vi "_UpdateUIDisplay.vi"(7 "Refs":T2, 9 "Action in":T1 caption="Action", 10 "Display State In in":T3 caption="State", 11 "Data In in":T6) -> (1 "Action out":T1 caption="Action", 2 "Display State In out":T3 caption="State", 3 "Data In out":T6)   [LabVIEW 2017, in "UI_TimeSelector.xctl"]
uses:
  UI_TimeSelector.xctl
  Data.ctl
  State.ctl
  Typedefs/INTERNAL-DATA.ctl
  Interface/DEF-Mode.ctl
  Typedefs/INTERNAL-REFs.ctl
  <vilib>/_xctls/Action.ctl
  <vilib>/_xctls/XControlSupport.lvlib
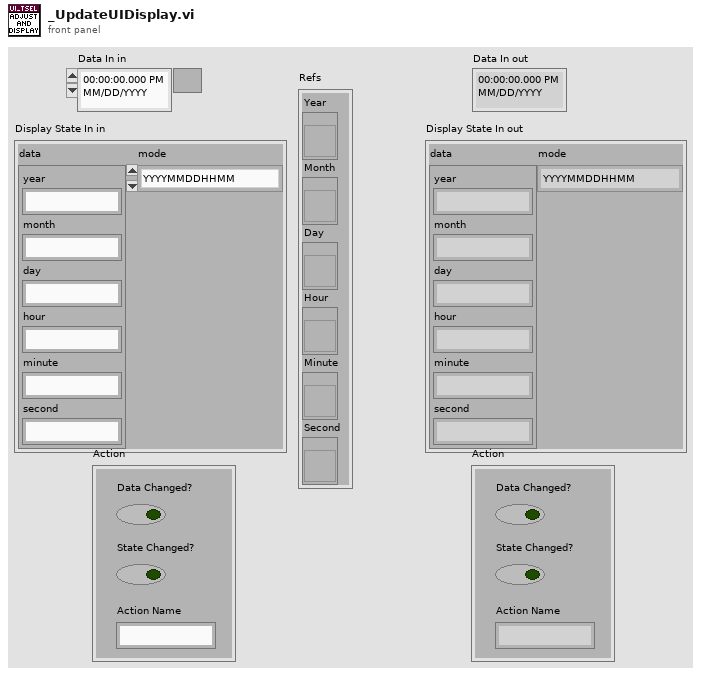
[diagram p1: front panel]
types:
  T1 = typedef "XControlSupport.lvlib/Action.ctl" = cluster{"Data Changed?":bool, "State Changed?":bool, "Action Name":string}
  T2 = typedef "UI_TimeSelector.xctl/INTERNAL-REFs.ctl" = cluster{"Year":refnum<vi>, "Month":refnum<vi>, "Day":refnum<vi>, "Hour":refnum<vi>, "Minute":refnum<vi>, "Second":refnum<vi>}
  T3 = typedef "UI_TimeSelector.xctl/State.ctl" = cluster{"data":T4, "mode":T5}
  T4 = typedef "UI_TimeSelector.xctl/INTERNAL-DATA.ctl" = cluster{"year":string, "month":string, "day":string, "hour":string, "minute":string, "second":string}
  T5 = typedef "UI_TimeSelector.xctl/DEF-Mode.ctl" = enum16{"YYYYMMDDHHMM", "YYYYMMDDHHMMSS", "YYYY", "YYYYMM", "YYYYMMDD", "HHMM", "HHMMSS"}
  T6 = typedef "UI_TimeSelector.xctl/Data.ctl" = timestamp
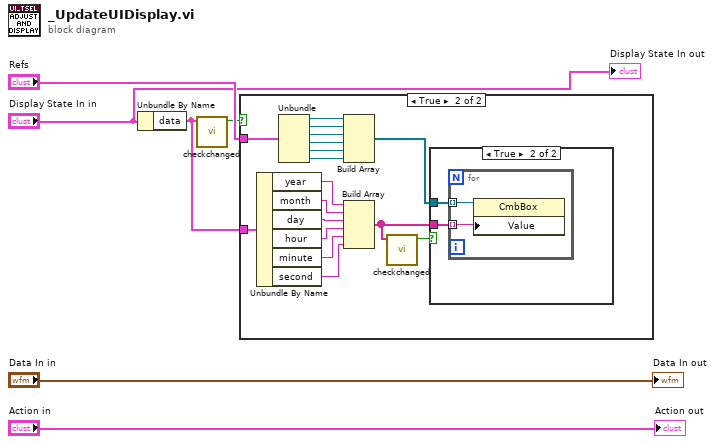
[diagram p0: block diagram]
diagram:
  n1 = Unbundle By Name("Display State In in") -> ("data"=w2:T4)
  n2 = call "checkchanged.vi"("mode"=w2) -> ("Boolean"=w5:bool)  [unwired: 10 in]
  n3 = case shown="True" w5 {
    tunnel: "Refs" -> [_ w23]
    tunnel: w2 -> [_ w7]
    frame False {
    }
    frame True {
      n4 = Unbundle By Name(w7) -> ("year"=w16:string, "month"=w15:string, "day"=w14:string, "hour"=w13:string, "minute"=w12:string, "second"=w11:string)
      n5 = Unbundle(w23) -> ("Year"=w22:refnum<vi>, "Month"=w21:refnum<vi>, "Day"=w20:refnum<vi>, "Hour"=w19:refnum<vi>, "Minute"=w18:refnum<vi>, "Second"=w17:refnum<vi>)
      n6 = Build Array(w22, w21, w20, w19, w18, w17) -> (w10:refnum<vi>[])
      n7 = Build Array(w16, w15, w14, w13, w12, w11) -> (w9:string[])
      n8 = call "checkchanged.vi"("mode"=w9) -> ("Boolean"=w8:bool)  [unwired: 10 in]
      n9 = case shown="True" w8 {
        tunnel: w10 -> [_ w25]
        tunnel: w9 -> [_ w24]
        frame False {
        }
        frame True {
          n10 = for {
            tunnel: w25 -> [w27] mode=indexing
            tunnel: w24 -> [w26] mode=indexing
            n11 = property class="CmbBox"(reference=w27, "Value"=w26) -> ()  [unwired: 1 in, 2 out]
          }
        }
      }
    }
  }
  "Data In out" <- "Data In in"
  "Display State In out" <- "Display State In in"
  "Action out" <- "Action in"
